vi "Test - Timer Module - Unpause Timer 1.vi"(8 "error in (no error)":errorcluster, 11 "Module ID":i32) -> (0 "error out":errorcluster, 2 "Final Timer":timestamp format="%^<%H:%M:%S%3u>T", 3 "Pass":bool)   [LabVIEW 2018]
doc: "_____\nCreated using Delacor QMH Event Scripter 4.1.0.76."
uses:
  Libraries/Timer Module/Timer Module.lvlib
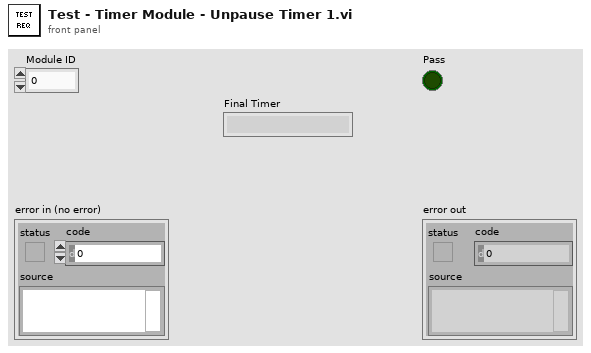
[diagram p1: front panel]
types:
  T1 = typedef "Timer Module.lvlib/Broadcast Events--cluster.ctl" = cluster{"Module Did Init":refnum<user-event>, "Status Updated":refnum<user-event>, "Error Reported":refnum<user-event>, "Module Did Stop":refnum<user-event>, "Update Module Execution Status":refnum<user-event>, "Timer Updated":refnum<user-event>}
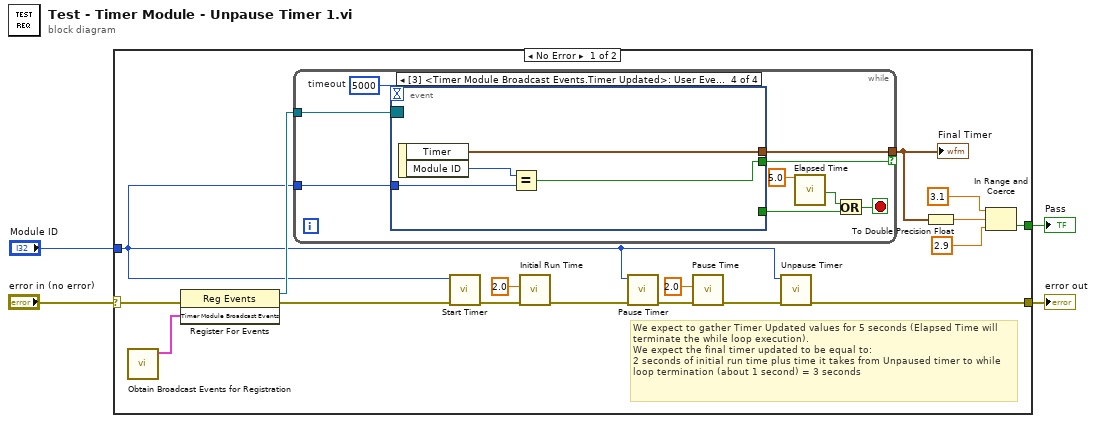
[diagram p0: block diagram]
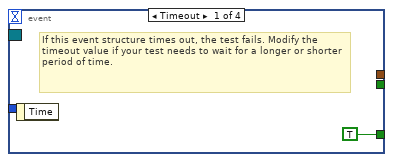
[diagram p2: hidden frame]
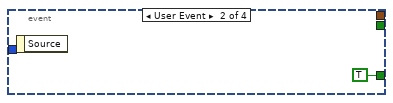
[diagram p3: hidden frame]
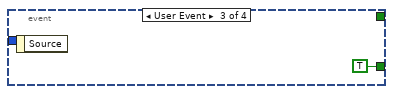
[diagram p4: hidden frame]
diagram:
  n1 = case shown="No Error" "error in (no error)" {
    selector: "error in (no error)" -> [w21 w38]
    tunnel: [w20 w38] -> w3
    tunnel: "Module ID" -> [w10 _]
    tunnel: [w5 _] -> w1
    frame No Error {
      # "We expect to gather Timer Updated values for 5 seconds (Elapsed Time will terminate the while loop execution). \nWe expect the final timer updated to be equal to:\n2 seconds of initial run time plus time it takes from Unpaused timer to while loop termination (about 1 second) = 3 seconds"
      n2 = call "Obtain Broadcast Events for Registration.vi"() -> ("Timer Module Broadcast Events"=w19:T1)  [unwired: 10 in, 1 out]
      n3 = register-events(error in=w21, w19) -> (reference out=w18:refnum<event-registration>, error out=w17:errorcluster)  [unwired: 1 in]
      n4 = while {
        tunnel: w18 -> [w30]
        tunnel: [w27] -> w9 if=w26
        tunnel: w10 -> [w22]
        stop <- w25 stop-if-true
        w29 = 5000  # timeout
        n5 = event shown="[3] <Timer Module Broadcast Events.Timer Updated>: User Event" {
          selector: w30 -> [_ _ _ _]
          dyn-events: _ -> [_ _ _ _]
          timeout: w29 -> [_ _ _ _]
          tunnel: [TRUE TRUE TRUE _] -> w28
          tunnel: [_ _ _ w37] -> w27
          tunnel: [_ _ _ w34] -> w26
          tunnel: w22 -> [_ _ _ w35]
          event Timeout {
            # "If this event structure times out, the test fails. Modify the timeout value if your test needs to wait for a longer or shorter period of time."
            n6 = event-data() -> ()  [unwired: 1 in, 1 out]
          }
          event User Event {
            n7 = event-data() -> ()  [unwired: 1 in, 1 out]
          }
          event User Event {
            n8 = event-data() -> ()  [unwired: 1 in, 1 out]
          }
          event User Event {
            n9 = event-data() -> ("Timer"=w37:timestamp, "Module ID"=w36:i32)  [unwired: 1 in]
            n10 = Equal?(x=w36, y=w35) -> (x = y?=w34:bool)
          }
        }
        n11 = call "Elapsed Time"("Time Target (s)"=5.0) -> ("Time has Elapsed"=w23:bool)  [unwired: 11 in, 7 out]
        n12 = Or(x=w23, y=w28) -> (x .or. y?=w25:bool)
      }
      "Final Timer" <- w9
      n13 = call "Start Timer.vi"("error in (no error)"=w17, "Module ID"=w10) -> ("error out"=w15:errorcluster)  [unwired: 9 in]
      n14 = call "Initial Run Time"("error in (no error)"=w15, "Delay Time (s)"=2.0) -> ("error out"=w14:errorcluster)  [unwired: 9 in]
      n15 = call "Pause Timer.vi"("error in (no error)"=w14, "Module ID"=w10) -> ("error out"=w12:errorcluster)  [unwired: 9 in]
      n16 = call "Pause Time"("error in (no error)"=w12, "Delay Time (s)"=2.0) -> ("error out"=w11:errorcluster)  [unwired: 9 in]
      n17 = call "Unpause Timer.vi"("error in (no error)"=w11, "Module ID"=w10) -> ("error out"=w20:errorcluster)  [unwired: 9 in]
      n18 = To Double Precision Float(number=w9) -> (double precision float=w8:dbl)
      n19 = In Range and Coerce(upper limit=3.1, x=w8, lower limit=2.9 ("upper limit")) -> (In Range?=w5:bool)  [unwired: 1 out]
    }
    frame Error {
    }
  }
  "error out" <- w3
  "Pass" <- w1
